vi "Actor Core.vi"(8 "error in":errorcluster, 11 "Actor in":refnum<class "Actor1_BasicNoLib_G4_4.0.0.lvclass">) -> (0 "error out":errorcluster, 3 "Actor out":refnum<class "Actor.lvclass">)   [LabVIEW 2020, in "Actor1_BasicNoLib_G4_4.0.0.lvclass"]
doc: "This is Actor Core.vi, the main message handling loop for Actors. An actor usually just sits in this loop and processes messages as they arrive. Any error returned by the message Do.vi call will stop the loop, with error code 43 as the cannonical signal to stop with no error sent to caller. Descendants may override that in Handle Error.vi."
uses:
  <resource>/Framework/Providers/Open_GDS/ClassProviders/ActorFramework/4.0.0/Actor1_BasicNoLib_G4_4.0.0/Actor1_BasicNoLib_G4_4.0.0_class/Actor1_BasicNoLib_G4_4.0.0.lvclass
  <vilib>/ActorFramework/Actor/Actor.lvclass
  C:/Program Files (x86)/National Instruments/LabVIEW 2020/vi.lib/ActorFramework/Actor/Actor.lvclass
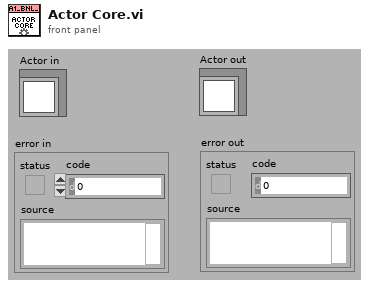
[diagram p1: front panel]
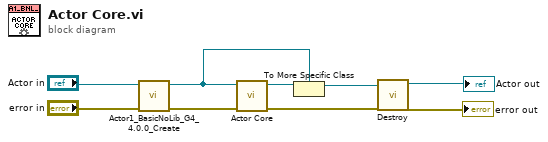
[diagram p0: block diagram]
diagram:
  n1 = call <resource>:"Actor1_BasicNoLib_G4_4.0.0_Create.vi"("error in (no error)"="error in", "reference in"="Actor in") -> ("error out"=w2:errorcluster, "reference out"=w3:refnum<class "Actor1_BasicNoLib_G4_4.0.0.lvclass">)  [unwired: 8 in]
  n2 = call-parent "Actor Core.vi"("error in"=w2, "Actor in"=w3) -> ("error out"=w1:errorcluster, "Actor out"=w7:refnum<class "Actor.lvclass">)  [unwired: 8 in]
  n3 = To More Specific Class(target class=w3, reference=w7) -> (specific class reference=w6:refnum<class "Actor1_BasicNoLib_G4_4.0.0.lvclass">)  [unwired: 1 in, 1 out]
  n4 = call-dynamic "Destroy.vi"("error in (no error)"=w1, "reference in"=w6) -> ("error out"=→"error out":errorcluster, "reference out"=→"Actor out":refnum<class "Actor1_BasicNoLib_G4_4.0.0.lvclass">)  [unwired: 8 in]
